vi "Abbreviate_string.vi"(0 "Input String":string, 1 "Max String Length":i32=50) -> (2 "Output String":string)   [LabVIEW 2010]
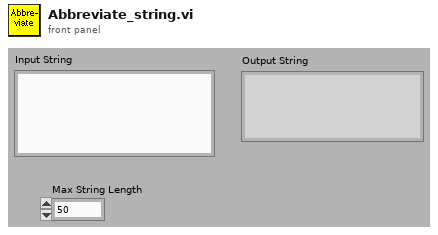
[diagram p1: front panel]
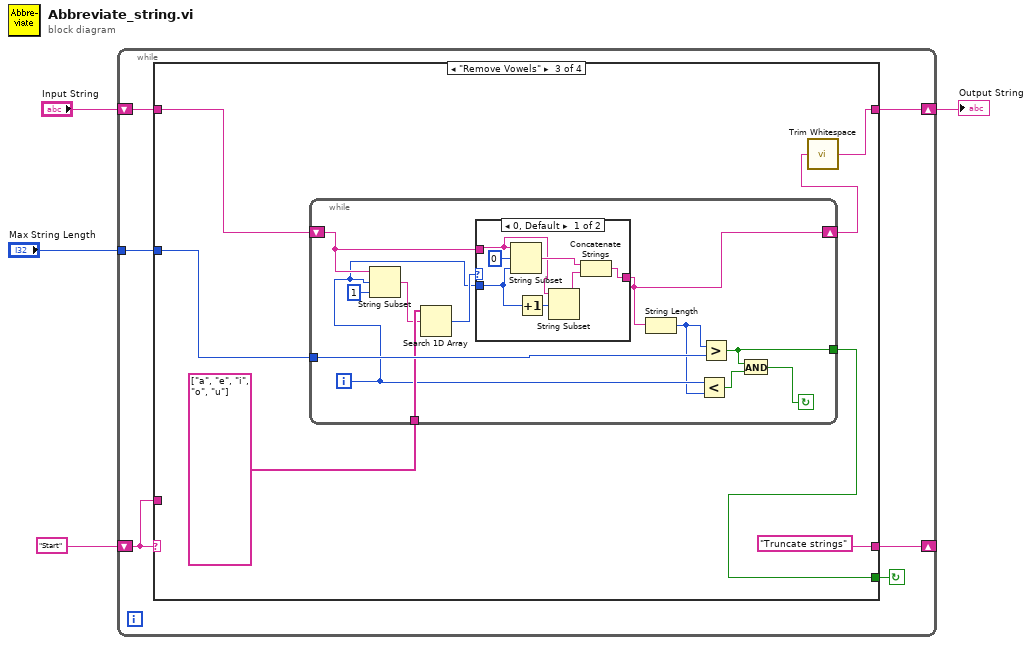
[diagram p0: block diagram]
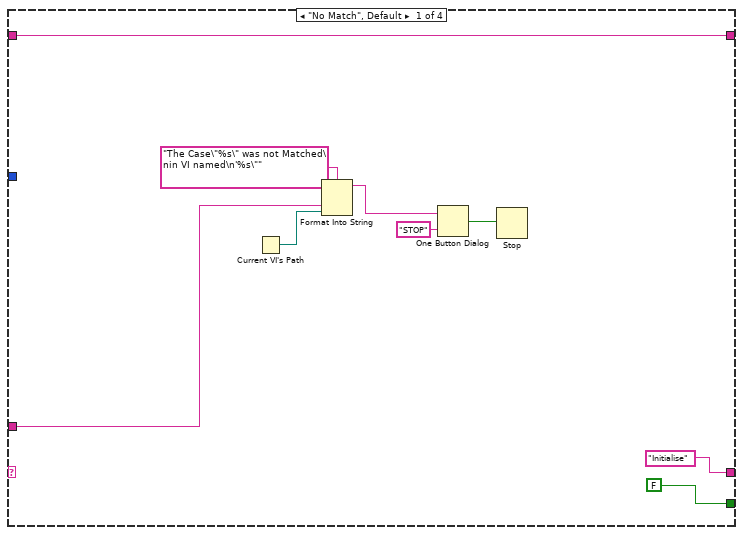
[diagram p2: hidden frame]
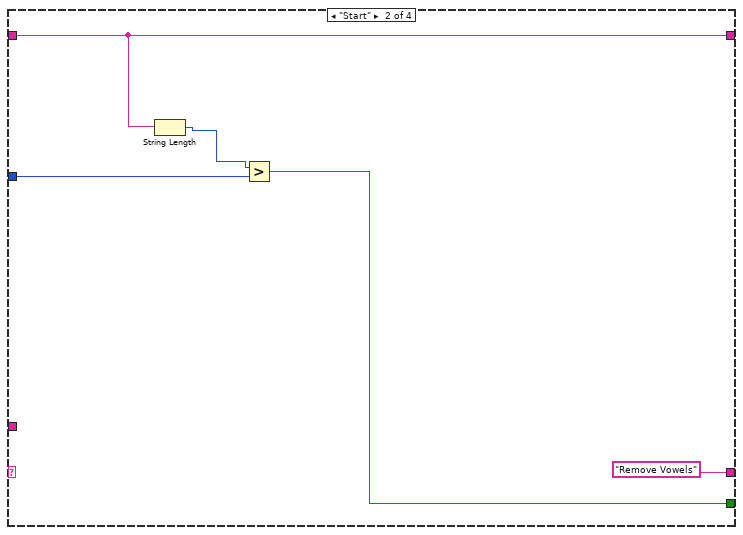
[diagram p3: hidden frame]
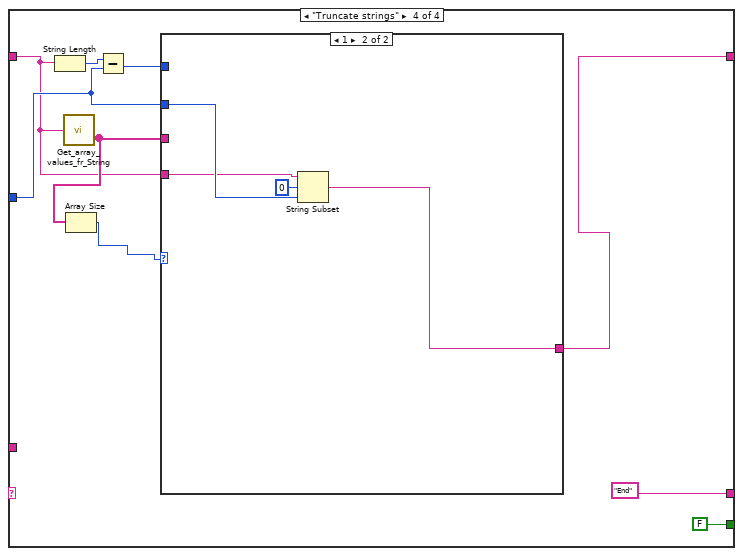
[diagram p5: hidden frame]
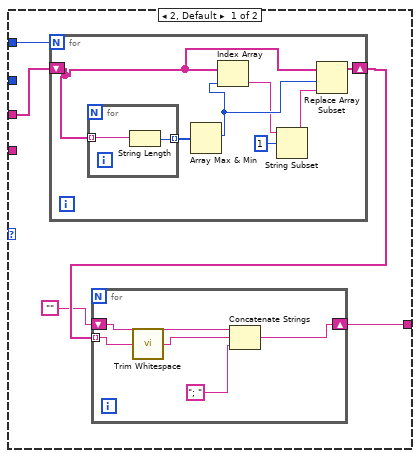
[diagram p6: hidden frame]
diagram:
  n1 = while {
    shift-left: "Start" -> [w8]
    shift-right: [w9] -> _
    shift-right: [w5] -> w3
    shift-left: "Input String" -> [w7]
    tunnel: "Max String Length" -> [w6]
    stop <- w10 continue-if-true
    n2 = case shown="\"Remove Vowels\"" w8 {
      tunnel: [FALSE w20 w29 FALSE] -> w10
      tunnel: ["Initialise" "Remove Vowels" "Truncate strings" "End"] -> w9
      tunnel: w8 -> [w14 _ _ _]
      tunnel: w7 -> [w11 w21 w28 w52]
      tunnel: w6 -> [_ w22 w30 w53]
      tunnel: [w11 w21 w25 w57] -> w5
      frame "No Match", Default {
        n3 = Current VI's Path() -> (path=w13:path)
        n4 = Format Into String(format string="The Case\"%s\" was not Matched\nin VI named\n'%s\"" ("Format String"), w14, w13) -> (resulting string=w17:string)  [unwired: 2 in, 1 out]
        n5 = One Button Dialog(message=w17, button name ("OK")="STOP") -> (true=w15:bool)
        n6 = Stop(stop? (T)=w15) -> ()
      }
      frame "Start" {
        n7 = String Length(string=w21) -> (length=w23:i32)
        n8 = Greater?(x=w23, y=w22) -> (0:w20:bool)
      }
      frame "Remove Vowels" {
        n9 = while {
          tunnel: w30 -> [w43]
          tunnel: [w40] -> w29
          shift-right: [w33] -> w26
          shift-left: w28 -> [w35]
          tunnel: string[] ["a", "e", "i", "o", "u"] ("appended array") -> [w38]
          i -> [w34]
          stop <- w41 continue-if-true
          n10 = String Subset(string=w35, offset (0)=w34, length (rest)=1 ("length (rest)")) -> (substring=w37:string)
          n11 = Search 1D Array(1D array=w38, element=w37) -> (index of element=w36:i32)  [unwired: 1 out]
          n12 = case shown="0, Default" w36 {
            tunnel: [w45 w51] -> w33
            tunnel: w35 -> [w44 w51]
            tunnel: w34 -> [w48 _]
            frame 0, Default {
              n13 = String Subset(string=w44, offset (0)=0, length (rest)=w48) -> (substring=w46:string)
              n14 = Increment(x=w48) -> (x+1=w49:i32)
              n15 = String Subset(string=w44, offset (0)=w49) -> (substring=w47:string)  [unwired: 1 out]
              n16 = Concatenate Strings(w46, w47) -> (w45:string)
            }
            frame -1 {
            }
          }
          n17 = String Length(string=w33) -> (length=w32:i32)
          n18 = Less?(x=w34, y=w32) -> (x < y?=w42:bool)
          n19 = Greater?(x=w32, y=w43) -> (0:w40:bool)
          n20 = And(x=w40, y=w42) -> (x .and. y?=w41:bool)
        }
        n21 = call <vilib>:"Trim Whitespace.vi"("string"=w26) -> ("trimmed string"=w25:string)  [unwired: 1 in]
      }
      frame "Truncate strings" {
        n22 = String Length(string=w52) -> (length=w59:i32)
        n23 = call "Get_array_values_fr_String.vi"("String Value"=w52) -> ("String array"=w55:string[])  [unwired: 1 out]
        n24 = Array Size(array=w55) -> (size(s)=w54:i32)
        n25 = Subtract(x=w59, y=w53) -> (x-y=w58:i32)
        n26 = case shown="1" w54 {
          tunnel: w58 -> [w65 _]
          tunnel: [w62 w80] -> w57
          tunnel: w55 -> [w61 _]
          tunnel: w53 -> [_ w83]
          tunnel: w52 -> [_ w81]
          frame 2, Default {
            n27 = for {
              N: w65 -> [_]
              shift-right: [w74] -> w64
              shift-left: w61 -> [w75]
              n28 = for {
                tunnel: w75 -> [w79] mode=indexing
                tunnel: [w78] -> w77 mode=indexing
                n29 = String Length(string=w79) -> (length=w78:i32)
              }
              n30 = Array Max & Min(array=w77) -> (max index (indices)=w76:i32)  [unwired: 3 out]
              n31 = Index Array(array=w75, index=w76) -> (element=w72:string)
              n32 = String Subset(string=w72, offset (0)=1) -> (substring=w71:string)  [unwired: 1 out]
              n33 = Replace Array Subset(array=w75, new element=w71, index=w76) -> (w74:string[])
            }
            n34 = for {
              shift-right: [w68] -> w62
              shift-left: "" -> [w70]
              tunnel: w64 -> [w67] mode=indexing
              n35 = call <vilib>:"Trim Whitespace.vi"("string"=w67) -> ("trimmed string"=w66:string)  [unwired: 1 in]
              n36 = Concatenate Strings(w70, w66, "; " ("string")) -> (w68:string)
            }
          }
          frame 1 {
            n37 = String Subset(string=w81, offset (0)=0, length (rest)=w83) -> (substring=w80:string)
          }
        }
      }
    }
  }
  "Output String" <- w3
